vi "Error_Handling.vi"(8 "error in (no error)":errorcluster, 11 "type of dialog (OK msg:1)":T1=1 items=["no dialog", "OK message", "continue or stop message", "OK message + warnings", "continue/stop + warnings"]) -> (0 "error out":errorcluster, 3 "error?":bool)   [LabVIEW 2011]
doc: "This VI utilizes the General Error Handler subVI to create custom errors that are more pertinent to the SRP\ntester platform. \n\nInputs:\n1. type of dialog: Lets the user specify the type of dialog box that opens during the current error (see General Error Handler sub VI). \n\nOutputs:\n1. error?: Boolean value of error (see General Error Handler sub VI)."
uses:
  <vilib>/Utility/error.llb/DialogType.ctl
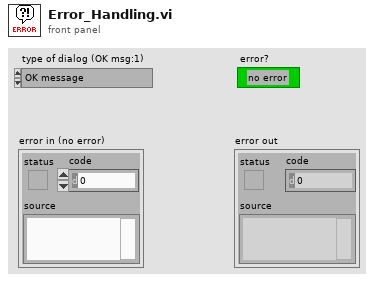
[diagram p1: front panel]
types:
  T1 = typedef "DialogType.ctl" = u16
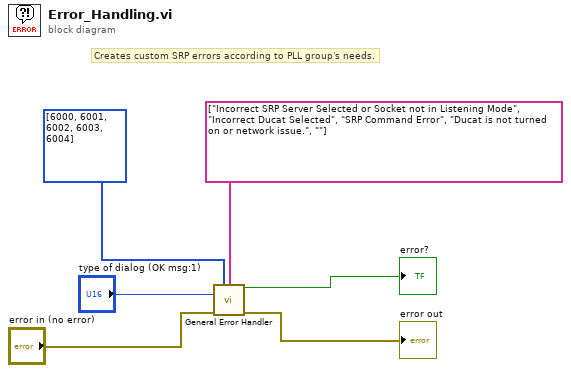
[diagram p0: block diagram]
diagram:
  # "Creates custom SRP errors according to PLL group's needs."
  n1 = call <vilib>:"General Error Handler.vi"("[user-defined codes]"=i32[] [6000, 6001, 6002, 6003, 6004], "[user-defined descriptions]"=string[] ["Incorrect SRP Server Selected or Socket not in Listening Mode", "Incorrect Ducat Selected", "SRP Command Error", "Ducat is not turned on or network issue.", ""], "type of dialog (OK msg:1)"="type of dialog (OK msg:1)", "error in (no error)"="error in (no error)") -> ("error?"=→"error?":bool, "error out"=→"error out":errorcluster)  [unwired: 7 in, 3 out]
